vi "Constants.vi"() -> ()   [LabVIEW 2015, in "J1939 Addon Shared.lvlib"]
uses:
  J1939 Addon Shared.lvlib
panel:
  in  "Refs.Incoming":string="IncomingData"
  in  "Refs.Outgoing":string="OutgoingData"
  in  "Refs.InternalResp":string="InternalResp"
  in  "Refs.InternalCmd":string="InternalCmd"
  in  "Protect Lamp":string="Protect Lamp"
  in  "Amber Warning":string="Amber Warning"
  in  "Red Stop":string="Red Stop"
  in  "Malfunction Indicator":string="Malfunction Indicator"
  in  "J1939 Monitor Settings":string="Monitor Settings"
  in  "Enable?":string="Enable"
  in  "SPN":string="SPN"
  in  "Occurrance":string="Occurrance"
  in  "FMI":string="FMI"
  in  "Simulation Page Name":string="Simulate"
  in  "Monitor Tool Page Name":string="Monitor"
  in  "DM2 Page Name":string="DM2 Previous DTCs"
  in  "DTC Page Name":string="DTC"
  in  "Simulated Diagnostics Page Name":string="Diagnostics"
  in  "Sim Device Page Name":string="Device"
  in  "DM1 Page Name":string="DM1 Active DTCs"
  in  "Simulation GUID":string="5d542ba3-f934-47c8-8526-922e6671f75c"
  in  "Monitor Tool GUID":string="ff8806fd-5187-43dd-8ad2-27d2e390b985"
  in  "DM2 GUID":string="a6e56184-1e6e-4172-a68a-86fd02f8cb1d"
  in  "DTC GUID":string="3533116e-8365-4b51-8f4f-44b0c5dae14b"
  in  "Simulated Diagnostics GUID":string="ab47f5e2-17b5-4786-91a9-aa1b83ce3202"
  in  "Sim Device GUID":string="a71bef71-deb0-46ee-be35-fd124c3f2929"
  in  "DM1 GUID":string="c2782be08-a048-47b9-a94e-6f4691487fca"
  in  "J1939 Compiled Settings":string="J1939 Compiled Settings"
  in  "Version":string="3.0.1"
  in  "RT Bitfile Location":path=path "c:/ni-rt/NIVeriStand/XNET"
  in  "RIO Device 986x":string="RIO Device 986x"
  in  "Enable 986x":string="Enable 986x"
  in  "Bitfile 986x":string="Bitfile 986x"
  in  "SPN Properties":string="SPN Properties"
  in  "Diagnostic Channel GUID":string="b62ef38f-3fa0-48a7-a2a3-2fe65e89e411"
  in  "DTC Clear Type":string="DTC Clear Type"
  in  "Requested DTC Status":string="Requested DTC Status"
  in  "# of DTCs Found":string="# of DTCs Found"
  in  "Address to Query":string="Address to Query"
  in  "Expected DTC":string="Expected DTC"
  in  "Diagnostic Command Status":string="Diagnostic Command Status"
  in  "Diagnostic Error Code":string="Diagnostic Error Code"
  in  "Diagnostic Command":string="Diagnostic Command"
  in  "Clear DTCs Page Name":string="Clear DTCs"
  in  "Clear DTCs GUID":string="5fe7a49a-076c-4c99-b5c3-65c554d9b468"
  in  "Verify DTCs Page Name":string="Verify DTC"
  in  "Verify DTCs GUID":string="a36e014a-9629-4cf0-b875-c21cd502bc82"
  in  "Diagnostics Page Name":string="Diagnostics"
  in  "Diagnostics GUID":string="fc9df2d5-46c1-45d0-98f7-1a68aab098d6"
  in  "Main Page GUID Disabled":string="A9661AD5-DF74-BF37-4CA8-5E0EF738F6FD"
  in  "Trigger Request":string="Trigger Request"
  in  "Request Destination":string="Request Destination"
  in  "Request PGN":string="Request PGN"
  in  "Request Section Name":string="Requests"
  in  "Debug Enable Name":string="Debug Enable"
  in  "Status Section Name":string="Status"
  in  "Transmit Properties":string="Transmit Properties"
  in  "Event Frame Page GUID":string="639C5D86-67C7-EF5B-B58A-94B163315B17"
  in  "Frame ID Name":string="ID"
  in  "J1939 XNET Settings":string="J1939 XNET Settings"
  in  "Outgoing Event Page Name":string="Event Triggered"
  in  "Outgoing Page Name":string="Outgoing"
  in  "Incoming Single Point Page Name":string="Single Point"
  in  "Incoming Page Name":string="Incoming"
  in  "Frame Page GUID":string="AA452EA6-A39D-713C-6D0F-1CFCE5C8BC25"
  in  "Signal Page GUID":string="FC3154D4-9B07-90D1-2A8F-6657A6DF127D"
  in  "Outgoing Event Page GUID":string="66CA57DF-0030-7FEB-7718-A68954D700B8"
  in  "Outgoing Page GUID":string="AF90FC7A-ACD0-CE24-9513-B991C453EC9C"
  in  "Incoming Single Point Page GUID":string="F09FE425-7E71-8634-77FE-097EFBD4E192"
  in  "Incoming Page GUID":string="AD3E1237-0B33-86CD-C074-2ECB9FA086C8"
  in  "Main Page GUID":string="5D441869-002F-93F2-B7E0-78053FA04717"
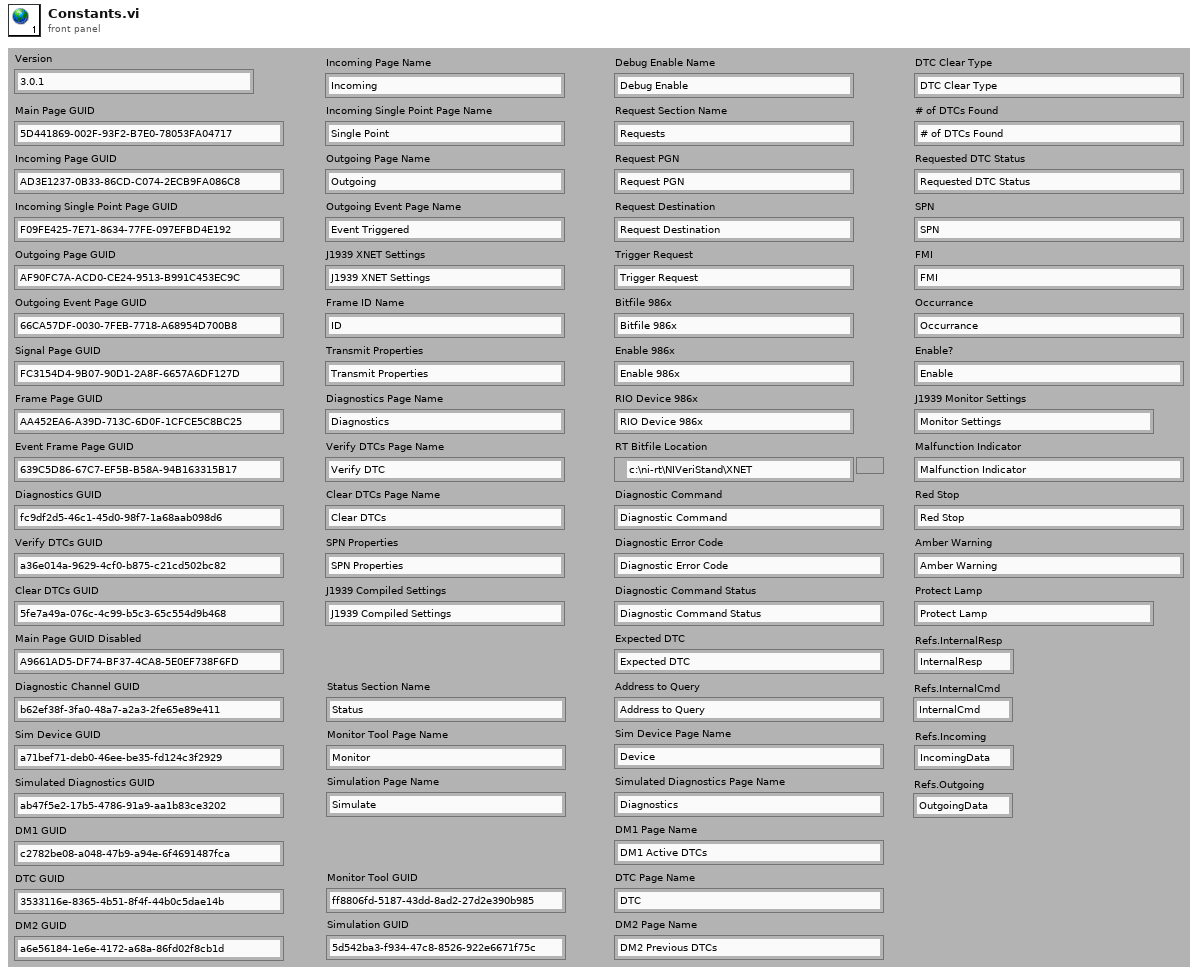
[diagram p1: front panel]
diagram:
